vi "etl.vi"() -> ()   [LabVIEW 2017]
panel:
  in  "stop 3":bool
  in  "mode":u16(ring) items=["usb", "analog"]
  in  "input 2":dbl min=-4.0 max=4.0 step=0.1 format="%1.2f"
  in  "stop 2":bool
  in  "lens 2":enum16{"0", "1"}(ring)=enum."1"
  in  "two lenses":bool
  in  "stop":bool
  in  "input":dbl min=-4.0 max=4.0 step=0.1 format="%1.2f"
  in  "lens":enum16{"0", "1"}(ring)
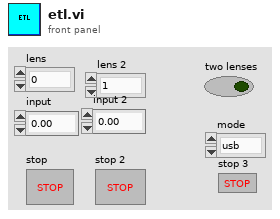
[diagram p1: front panel]
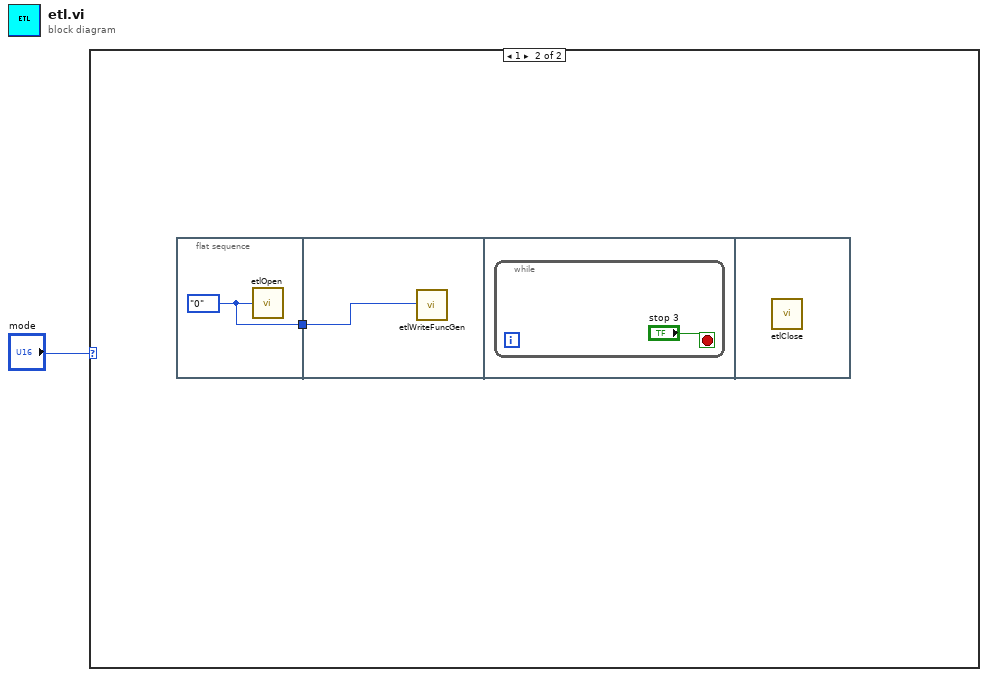
[diagram p0: block diagram]
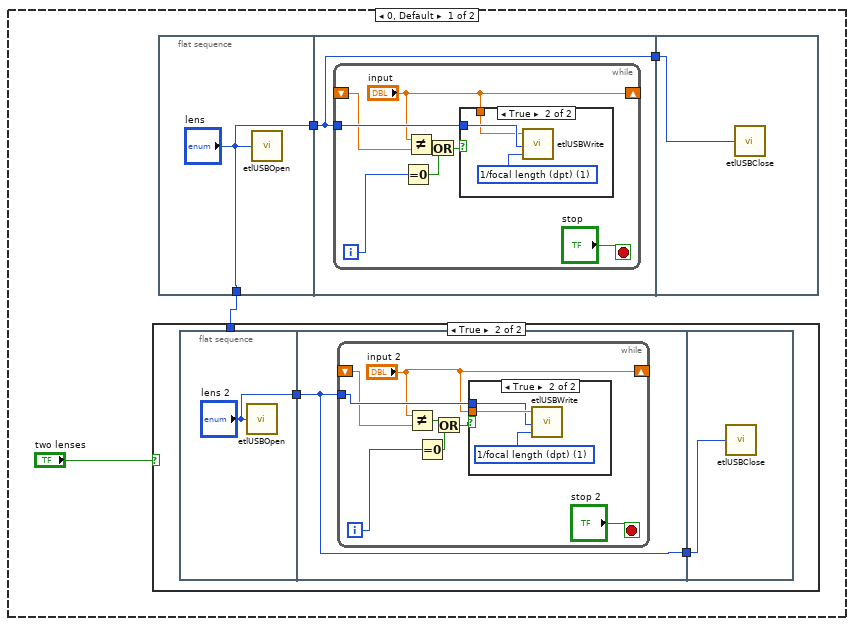
[diagram p2: hidden frame]
diagram:
  n1 = case shown="1" "mode" {
    frame 0, Default {
      n2 = case shown="True" "two lenses" {
        tunnel: w2 -> [_ _]
        frame False {
        }
        frame True {
          n3 = flat-sequence {
            tunnel: ["lens 2"] -> w7
            tunnel: w7 -> [w9]
            tunnel: [w9] -> w6
            tunnel: w6 -> [w21]
            frame #0 {
              n4 = call "etlUSBOpen.vi"("lens"="lens 2") -> ()  [unwired: 1 in, 1 out]
            }
            frame #1 {
              n5 = while {
                tunnel: w9 -> [w16]
                shift-right: ["input 2"] -> _
                shift-left: _ -> [w14]
                i -> [w10]
                stop <- "stop 2" stop-if-true
                n6 = Not Equal?(x="input 2", y=w14) -> (x != y?=w13:bool)
                n7 = Equal To 0?(x=w10) -> (x = 0?=w11:bool)
                n8 = Or(x=w13, y=w11) -> (x .or. y?=w12:bool)
                n9 = case shown="True" w12 {
                  tunnel: "input 2" -> [_ w19]
                  tunnel: w16 -> [_ w18]
                  frame False {
                  }
                  frame True {
                    w20 = u16 1 items=["position (um)", "1/focal length (dpt)"] ("mode")
                    n10 = call "etlUSBWrite.vi"("mode"=w20, "lens"=w18, "input"=w19) -> ()  [unwired: 1 in]
                  }
                }
              }
            }
            frame #2 {
              n11 = call "etlUSBClose.vi"("lens"=w21) -> ()  [unwired: 1 in]
            }
          }
        }
      }
      n12 = flat-sequence {
        tunnel: ["lens"] -> w5
        tunnel: ["lens"] -> w2
        tunnel: w5 -> [w23]
        tunnel: [w23] -> w4
        tunnel: w4 -> [w35]
        frame #0 {
          n13 = call "etlUSBOpen.vi"("lens"="lens") -> ()  [unwired: 1 in, 1 out]
        }
        frame #1 {
          n14 = while {
            tunnel: w23 -> [w31]
            shift-right: ["input"] -> _
            shift-left: _ -> [w28]
            i -> [w24]
            stop <- "stop" stop-if-true
            n15 = Equal To 0?(x=w24) -> (x = 0?=w25:bool)
            n16 = Not Equal?(x="input", y=w28) -> (x != y?=w27:bool)
            n17 = Or(x=w27, y=w25) -> (x .or. y?=w26:bool)
            n18 = case shown="True" w26 {
              tunnel: w31 -> [_ w34]
              tunnel: "input" -> [_ w32]
              frame False {
              }
              frame True {
                w33 = u16 1 items=["position (um)", "1/focal length (dpt)"] ("mode")
                n19 = call "etlUSBWrite.vi"("mode"=w33, "lens"=w34, "input"=w32) -> ()  [unwired: 1 in]
              }
            }
          }
        }
        frame #2 {
          n20 = call "etlUSBClose.vi"("lens"=w35) -> ()  [unwired: 1 in]
        }
      }
    }
    frame 1 {
      n21 = flat-sequence {
        tunnel: [w37] -> w36
        tunnel: w36 -> [w38]
        frame #0 {
          w37 = enum16{"0", "1"}."0" ("lens")
          n22 = call "etlOpen.vi"("lens"=w37) -> ()  [unwired: 1 in]
        }
        frame #1 {
          n23 = call "etlWriteFuncGen.vi"("lens"=w38) -> ()  [unwired: 1 in]
        }
        frame #2 {
          n24 = while {
            stop <- "stop 3" stop-if-true
          }
        }
        frame #3 {
          n25 = call "etlClose.vi"() -> ()  [unwired: 2 in]
        }
      }
    }
  }
